vi "EOL Check AP Vent Limits.vi"(7 "Pass? In":bool=TRUE, 8 "Error Table":string[][](array[string]), 10 "Sun Shade Close Force":T1 {"Truncation End" format="%.2g"; "Truncation Start" format="%.2g"; "Overall Max" format="%.2g"; "Overall Min" format="%.2g"}, 11 "Vent Force Calculated Data":dbl) -> (0 "Error Table 2":string[][](array[string]), 2 "Vent Force Data and Limits":dbl[](array[numeric]), 3 "Pass?":bool)   [LabVIEW 2018]
uses:
  05.UserVI's/type defs/Vent AP Limts Seq.ctl
panel:
  # "Start"
  # "Min"
  # "N"
  # "End"
  # "Max"
  # "N"
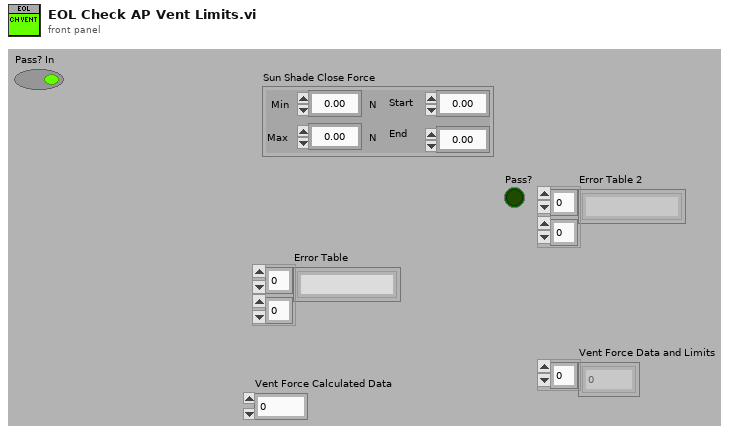
[diagram p1: front panel]
types:
  T1 = typedef "Vent AP Limts Seq.ctl" = cluster{"Overall Min":dbl, "Overall Max":dbl, "Truncation Start":dbl, "Truncation End":dbl}
  T2 = cluster{"Vent Force Calculated Data":dbl, "Sun Shade Close Force":T1, "Error Table":string[][], "Pass? In":bool}
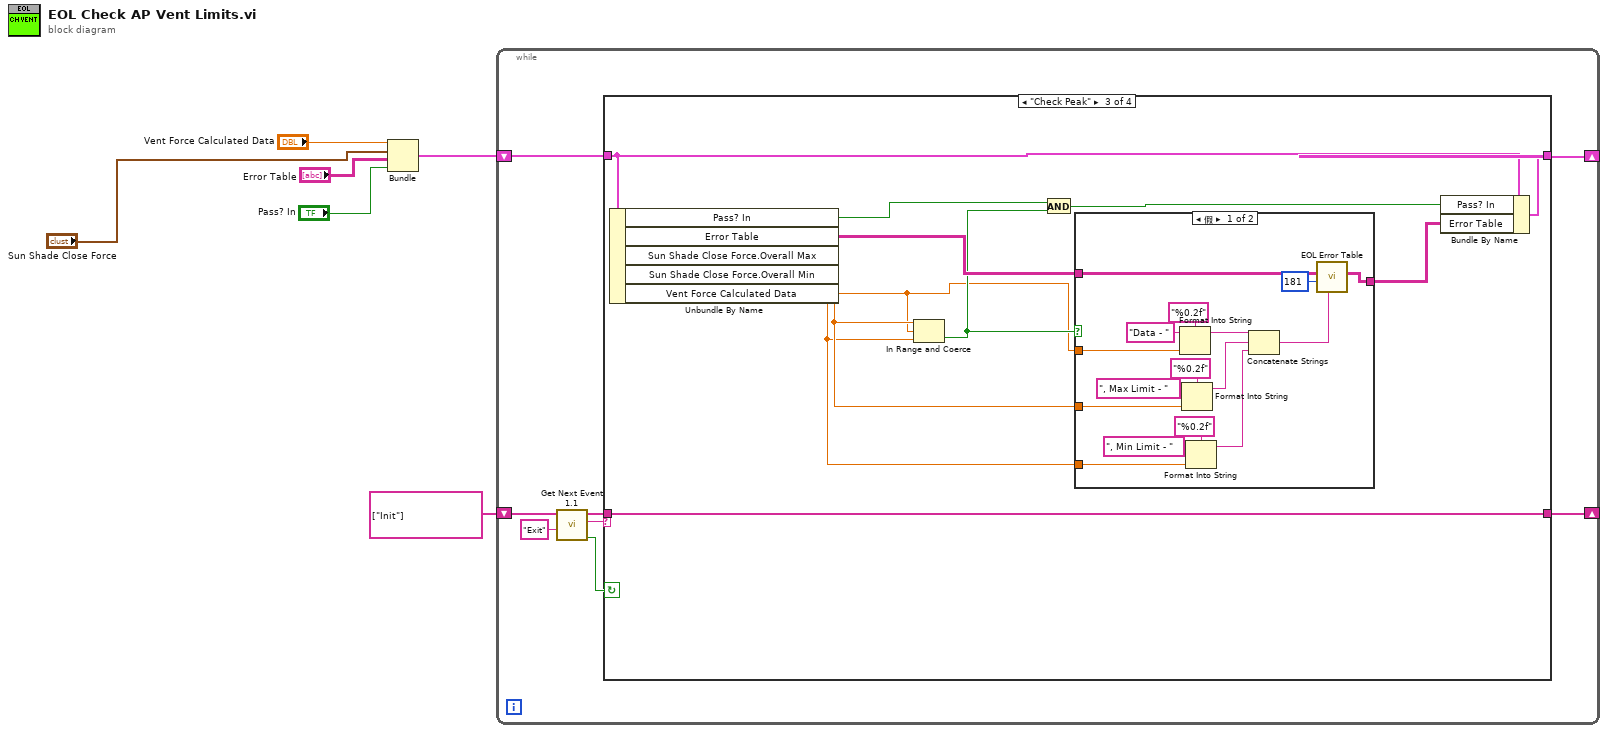
[diagram p0: block diagram]
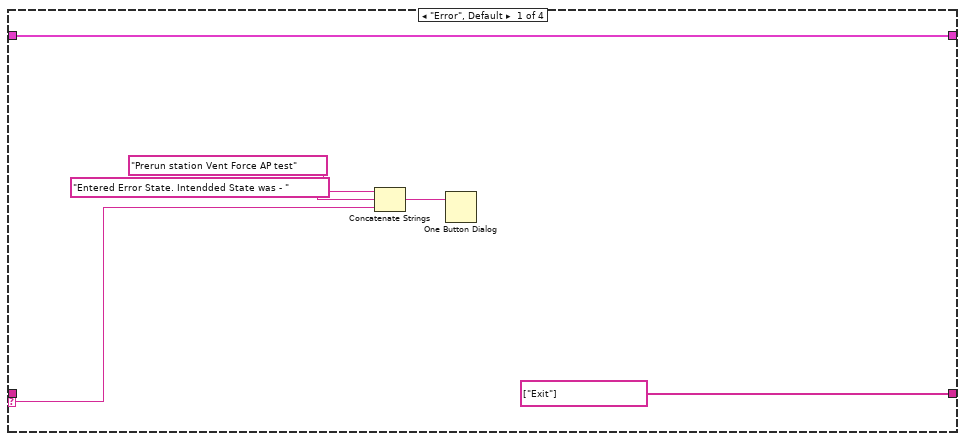
[diagram p2: hidden frame]
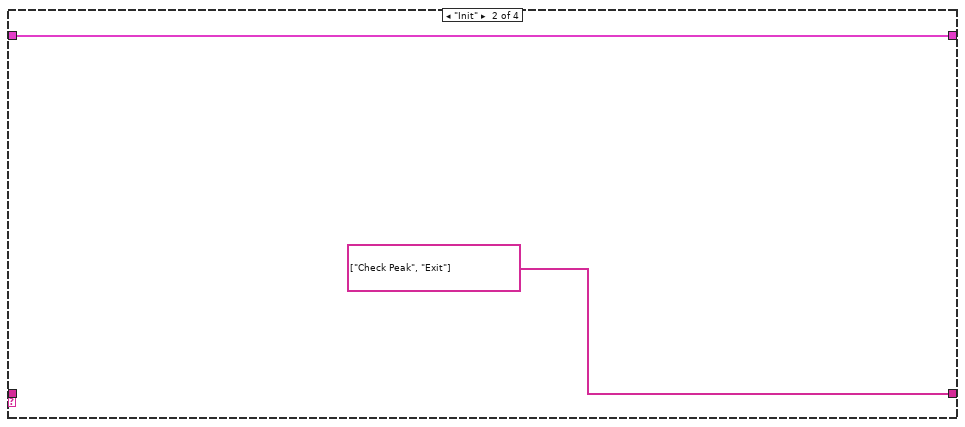
[diagram p3: hidden frame]
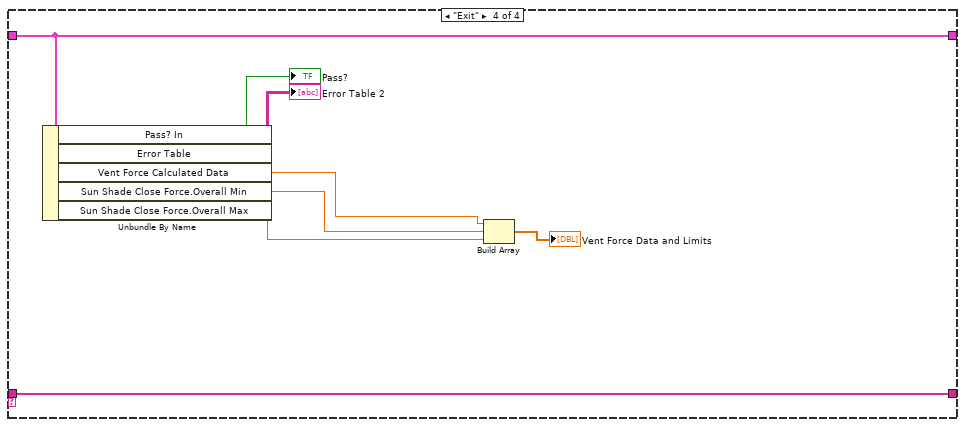
[diagram p5: hidden frame]
diagram:
  n1 = Bundle("Vent Force Calculated Data"="Vent Force Calculated Data", "Sun Shade Close Force"="Sun Shade Close Force", "Error Table"="Error Table", "Pass? In"="Pass? In") -> (w4:T2)  [unwired: 1 in]
  n2 = while {
    shift-right: [w10] -> _
    shift-left: string[] ["Init"] ("event queue out") -> [w9]
    shift-right: [w7] -> _
    shift-left: w4 -> [w8]
    stop <- w13 continue-if-true
    n3 = call "Get Next Event 1.1.vi"("Exit Event"="Exit", "event queue in"=w9) -> ("Condition (Exit:F)"=w13:bool, "next event"=w14:string, "event queue out"=w11:string[])  [unwired: 6 in, 1 out]
    n4 = case shown="\"Check Peak\"" w14 {
      selector: w14 -> [w16 _ _ _]
      tunnel: w11 -> [_ _ w28 w58]
      tunnel: [string[] ["Exit"] ("event queue out") string[] ["Check Peak", "Exit"] ("event queue out") w28 w58] -> w10
      tunnel: w8 -> [w15 w22 w32 w57]
      tunnel: [w15 w22 w29 w57] -> w7
      frame "Error", Default {
        n5 = Concatenate Strings("Prerun station Vent Force AP test" ("string"), "Entered Error State. Intendded State was - " ("string"), w16) -> (w19:string)
        n6 = One Button Dialog(message=w19) -> ()  [unwired: 1 in, 1 out]
      }
      frame "Init" {
      }
      frame "Check Peak" {
        n7 = Unbundle By Name(w32) -> ("Pass? In"=w31:bool, "Error Table"=w33:string[][], "Sun Shade Close Force.Overall Max"=w26:dbl, "Sun Shade Close Force.Overall Min"=w24:dbl, "Vent Force Calculated Data"=w23:dbl)
        n8 = In Range and Coerce(upper limit=w26, x=w23, lower limit=w24) -> (In Range?=w25:bool)  [unwired: 1 out]
        n9 = And(x=w31, y=w25) -> (x .and. y?=w30:bool)
        n10 = case shown="假" w25 {
          tunnel: w33 -> [w49 w50]
          tunnel: w26 -> [w46 _]
          tunnel: [w35 w50] -> w27
          tunnel: w23 -> [w41 _]
          tunnel: w24 -> [w38 _]
          frame False {
            n11 = Format Into String(format string="%0.2f", initial string="Data - ", w41) -> (resulting string=w43:string)  [unwired: 1 in, 1 out]
            n12 = Format Into String(format string="%0.2f", initial string=", Max Limit - ", w46) -> (resulting string=w42:string)  [unwired: 1 in, 1 out]
            n13 = Format Into String(format string="%0.2f", initial string=", Min Limit - ", w38) -> (resulting string=w37:string)  [unwired: 1 in, 1 out]
            n14 = Concatenate Strings(w43, w42, w37) -> (w36:string)
            n15 = call "EOL Error Table.vi"("Error Description"=w36, "Error No."=u16 181, "Error Table In"=w49) -> ("Error Table Out"=w35:string[][])  [unwired: 7 in, 1 out]
          }
          frame True {
          }
        }
        n16 = Bundle By Name(cluster=w32, "Pass? In"=w30, "Error Table"=w27) -> (w29:T2)
      }
      frame "Exit" {
        n17 = Unbundle By Name(w57) -> ("Pass? In"=→"Pass?":bool, "Error Table"=→"Error Table 2":string[][], "Vent Force Calculated Data"=w52:dbl, "Sun Shade Close Force.Overall Min"=w54:dbl, "Sun Shade Close Force.Overall Max"=w51:dbl)
        n18 = Build Array(w52, w54, w51) -> (→"Vent Force Data and Limits":dbl[])
      }
    }
  }
